vi "getStateNamesByChannel.vi"(8 "error in (no error)":errorcluster, 10 "channel_name":string, 11 "ChannelArray in":refnum<class "ChannelArray.lvclass">) -> (0 "error out":errorcluster, 2 "state_names":string[](array[string]), 3 "ChannelArray out":refnum<class "ChannelArray.lvclass">)   [LabVIEW 2011, in "Tools.lvlib" / "DatabaseHelpers.lvlib" / "ChannelArray.lvclass"]
uses:
  ChannelArray.lvclass
  Channel/Channel.lvclass
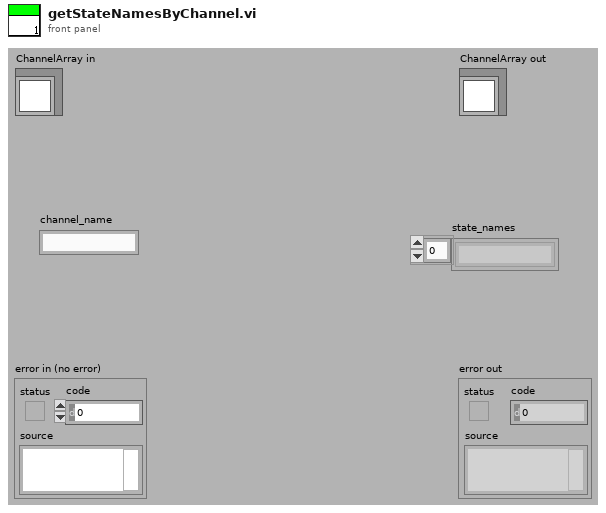
[diagram p1: front panel]
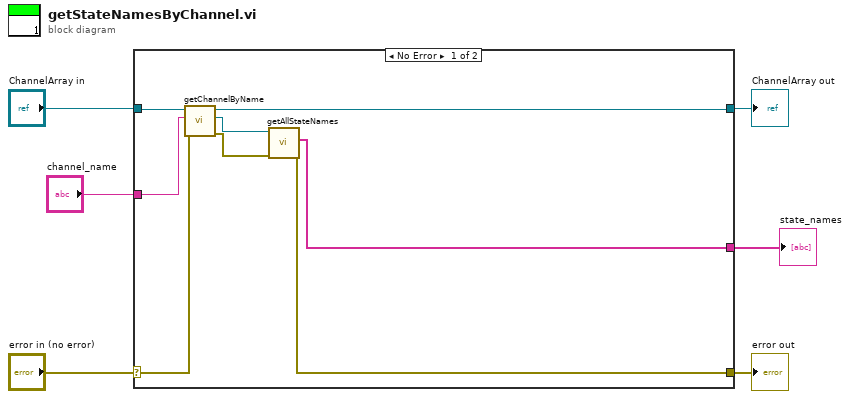
[diagram p0: block diagram]
diagram:
  n1 = case shown="No Error" "error in (no error)" {
    selector: "error in (no error)" -> [w12 w16]
    tunnel: [w7 w16] -> w5
    tunnel: [w8 w15] -> w3
    tunnel: "ChannelArray in" -> [w14 w15]
    tunnel: "channel_name" -> [w13 _]
    tunnel: [w10 _] -> w1
    frame No Error {
      n2 = call-dynamic "getChannelByName.vi"("error in (no error)"=w12, "channel_name"=w13, "ChannelArray in"=w14) -> ("error out"=w9:errorcluster, "Channel"=w11:refnum<class "Channel.lvclass">, "ChannelArray out"=w8:refnum<class "ChannelArray.lvclass">)  [unwired: 5 in, 1 out]
      n3 = call-dynamic "getAllStateNames.vi"("error in (no error)"=w9, "Channel in"=w11) -> ("error out"=w7:errorcluster, "state_names"=w10:string[])  [unwired: 7 in, 1 out]
    }
    frame Error {
    }
  }
  "error out" <- w5
  "ChannelArray out" <- w3
  "state_names" <- w1
